vi "Background Loop Step.vi"(8 "error in (no error)":errorcluster, 10 "Action":T1, 11 "Instrument Actor in":refnum<class "Instrument Actor.lvclass">) -> (0 "error out":errorcluster, 1 "Next step delay":i32, 2 "Action out":T1=enum."Stop", 3 "Instrument Actor out":refnum<class "Instrument Actor.lvclass">, 4 "Result":refnum<class "Acquired Result.lvclass">)   [LabVIEW 2021, in "Instrument Actor.lvclass"]
uses:
  Instrument Actor.lvclass
  Worker/Worker Actor/Background Loop Action.ctl
  NHMFL_Core/Libraries/Instruments/Results/Acquired Result/Acquired Result.lvclass
  Instrument Actor.lvclass/Instrument Actor.ctl
  Read Instrument driver.vi
  Write Instrument driver.vi
  NHMFL_Core/Libraries/Instruments/Instrument Driver/Instrument Driver.lvclass
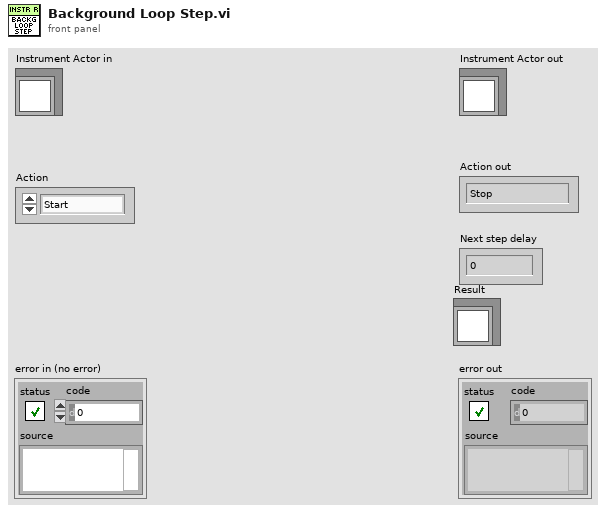
[diagram p1: front panel]
types:
  T1 = typedef "Background Loop Action.ctl" = enum16{"Start", "Continue", "Stop"}
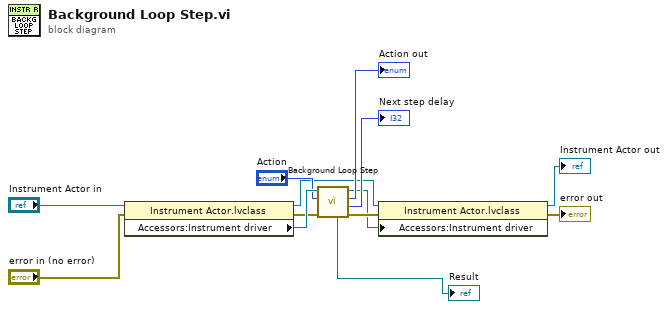
[diagram p0: block diagram]
diagram:
  n1 = property class="Instrument Actor.lvclass"(reference="Instrument Actor in", error in="error in (no error)") -> (reference out=w5:refnum<class "Instrument Actor.lvclass">, error out=w8:errorcluster, "Accessors:Instrument driver"=w12:refnum<class "Instrument Driver.lvclass">)
  n2 = call-dynamic "Background Loop Step.vi"("error in (no error)"=w8, "Action"="Action", "Instrument Driver in"=w12) -> ("error out"=w7:errorcluster, "Next step delay"=→"Next step delay":i32, "Action out"=→"Action out":T1, "Instrument Driver out"=w6:refnum<class "Instrument Driver.lvclass">, "Result"=→"Result":refnum<class "Acquired Result.lvclass">)  [unwired: 4 in]
  n3 = property class="Instrument Actor.lvclass"(reference=w5, error in=w7, "Accessors:Instrument driver"=w6) -> (reference out=→"Instrument Actor out":refnum<class "Instrument Actor.lvclass">, error out=→"error out":errorcluster)
